vi "Main.vi"() -> ()   [LabVIEW 2022 SP3]
doc: "Use this template to build a producer/consumer design pattern with events to produce queue items. Use this design pattern instead of the User Interface Event Handler pattern for user interfaces when you want to execute code asynchronously in response to an event without slowing the user interface responsiveness."
uses:
  MainBuf.ctl
  ed44cc61-03a2-4c3f-bcab-11a29ff6dbea.vi
  <vilib>/measure/NI_MABase.lvlib
panel:
  in  "Setup":bool
  out "Waveform Graph":waveform(dbl)(graph)
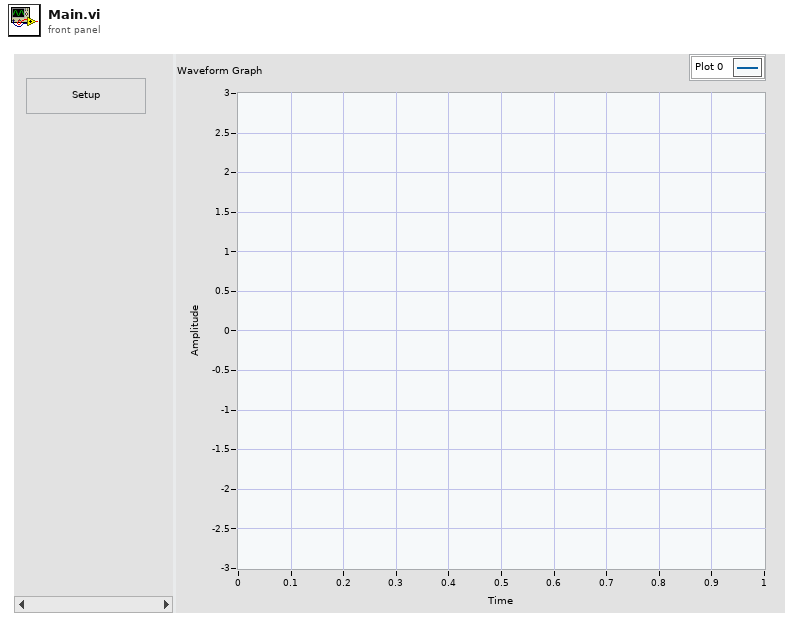
[diagram p1: front panel]
types:
  T1 = typedef "MainBuf.ctl" = cluster{"signal type":enum16{"Sine Wave", "Triangle Wave", "Square Wave", "Sawtooth Wave"}, "frequency":dbl, "amplitude":dbl, "phase":dbl, "offset":dbl, "square wave duty cycle (%)":dbl, "sampling info":cluster{"Fs":dbl, "#s":dbl}, "Reset":bool}
  T2 = enum16{"Sine Wave", "Triangle Wave", "Square Wave", "Sawtooth Wave"}
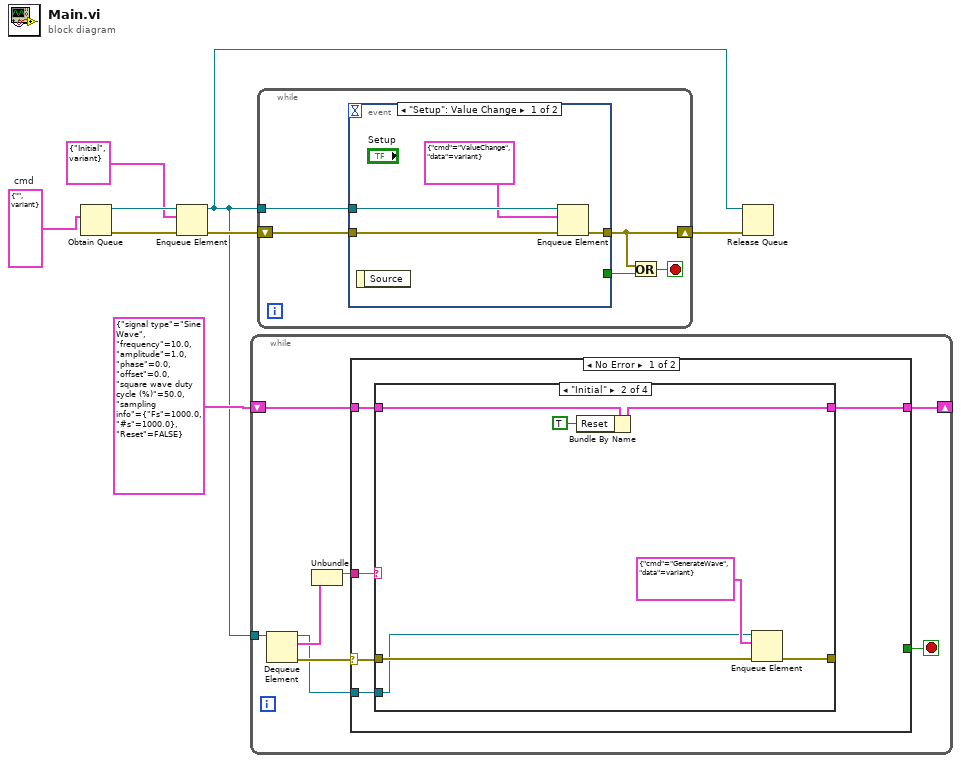
[diagram p0: block diagram]
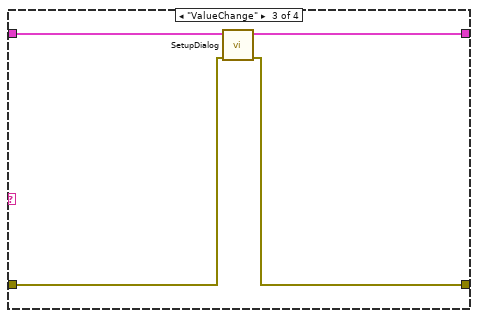
[diagram p3: hidden frame]
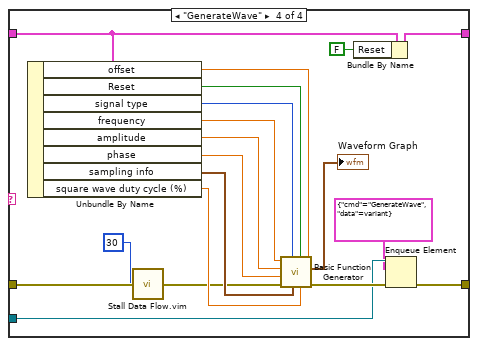
[diagram p4: hidden frame]
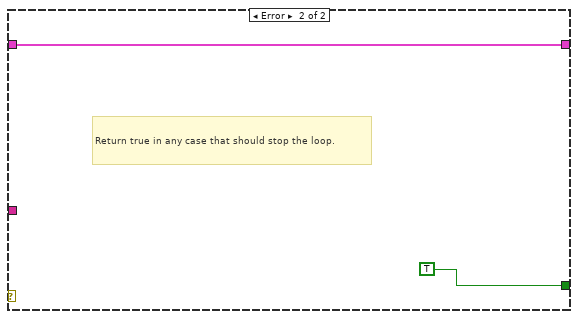
[diagram p5: hidden frame]
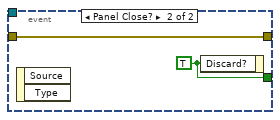
[diagram p6: hidden frame]
diagram:
  w6 = cluster{"cmd":string, "data":variant} {"cmd"="", "data"=variant}  # cmd
  n1 = Obtain Queue(element data type=w6) -> (queue out=w3:refnum<queue>, error out=w8:errorcluster)  [unwired: 4 in, 1 out]
  n2 = Enqueue Element(queue=w3, element=cluster{"cmd":string, "data":variant} {"cmd"="Initial", "data"=variant}, error in (no error)=w8) -> (queue out=w2:refnum<queue>, error out=w4:errorcluster)  [unwired: 1 in, 1 out]
  n3 = while {
    tunnel: w2 -> [w16]
    shift-right: [w11] -> _
    shift-left: T1 {"signal type"=enum."Sine Wave", "frequency"=10.0, "amplitude"=1.0, "phase"=0.0, "offset"=0.0, "square wave duty cycle (%)"=50.0, "sampling info"={"Fs"=1000.0, "#s"=1000.0}, "Reset"=FALSE} -> [w10]
    stop <- w13 stop-if-true
    n4 = Dequeue Element(queue=w16) -> (queue out=w9:refnum<queue>, element=w14:cluster{"cmd":string, "data":variant}, error out=w15:errorcluster)  [unwired: 2 in, 1 out]
    n5 = Unbundle(w14) -> ("cmd"=w12:string)  [unwired: 1 out]
    n6 = case shown="No Error" w15 {
      selector: w15 -> [w19 _]
      tunnel: w12 -> [w18 _]
      tunnel: [_ TRUE] -> w13
      tunnel: [w20 w54] -> w11
      tunnel: w10 -> [w21 w54]
      tunnel: w9 -> [w17 _]
      frame No Error {
        n7 = case shown="\"Initial\"" w18 {
          tunnel: w21 -> [w23 w30 w33 w53]
          tunnel: [w23 w26 w32 w38] -> w20
          tunnel: w19 -> [w22 w29 w34 w44]
          tunnel: [w22 w28 w31 w42] -> _
          tunnel: w17 -> [_ w24 _ w41]
          frame Default {
          }
          frame "Initial" {
            n8 = Bundle By Name(cluster=w30, "Reset"=TRUE) -> (w26:T1)
            n9 = Enqueue Element(queue=w24, element=cluster{"cmd":string, "data":variant} {"cmd"="GenerateWave", "data"=variant}, error in (no error)=w29) -> (error out=w28:errorcluster)  [unwired: 1 in, 2 out]
          }
          frame "ValueChange" {
            n10 = call "SetupDialog.vi"("error in (no error)"=w34, "Cluster in"=w33) -> ("error out"=w31:errorcluster, "Cluster out"=w32:T1)  [unwired: 8 in]
          }
          frame "GenerateWave" {
            n11 = Unbundle By Name(w53) -> ("offset"=w48:dbl, "Reset"=w47:bool, "signal type"=w52:T2, "frequency"=w51:dbl, "amplitude"=w50:dbl, "phase"=w49:dbl, "sampling info"=w46:cluster{"Fs":dbl, "#s":dbl}, "square wave duty cycle (%)"=w45:dbl)
            n12 = call "Stall Data Flow.vim"("value in"=w44, "milliseconds to wait"=u32 30) -> ("value out"=w36:errorcluster)  [unwired: 1 out]
            n13 = call <vilib>:"Basic Function Generator.vi"("offset"=w48, "square wave duty cycle (%)"=w45, "reset signal"=w47, "sampling info"=w46, "signal type"=w52, "error in (no error)"=w36, "phase"=w49, "amplitude"=w50, "frequency"=w51) -> ("error out"=w43:errorcluster, "signal out"=→"Waveform Graph":waveform(dbl))  [unwired: 1 out]
            n14 = Bundle By Name(cluster=w53, "Reset"=FALSE) -> (w38:T1)
            n15 = Enqueue Element(queue=w41, element=cluster{"cmd":string, "data":variant} {"cmd"="GenerateWave", "data"=variant}, error in (no error)=w43) -> (error out=w42:errorcluster)  [unwired: 1 in, 2 out]
          }
        }
      }
      frame Error {
        # "Return true in any case that should stop the loop."
      }
    }
  }
  n16 = while {
    shift-right: [w56] -> w7
    shift-left: w4 -> [w59]
    tunnel: w2 -> [w60]
    stop <- w57 stop-if-true
    n17 = event shown="[0] \"Setup\": Value Change" {
      selector: _ -> [_ _]
      dyn-events: _ -> [_ _]
      timeout: _ -> [_ _]
      tunnel: w60 -> [w64 _]
      tunnel: w59 -> [w63 w66]
      tunnel: [w62 w66] -> w56
      tunnel: [_ w65] -> w58
      event "Setup": Value Change {
        n18 = event-data() -> ()  [unwired: 1 in, 1 out]
        n19 = Enqueue Element(queue=w64, element=cluster{"cmd":string, "data":variant} {"cmd"="ValueChange", "data"=variant}, error in (no error)=w63) -> (error out=w62:errorcluster)  [unwired: 1 in, 2 out]
      }
      event Panel Close? {
        w65 = TRUE ("Discard?")
        n20 = event-data() -> ()  [unwired: 1 in, 2 out]
        n21 = event-data("Discard?"=w65) -> ()  [unwired: 1 in, 1 out]
      }
    }
    n22 = Or(x=w56, y=w58) -> (x .or. y?=w57:bool)
  }
  n23 = Release Queue(queue=w2, error in (no error)=w7) -> ()  [unwired: 1 in, 3 out]
